vi "Stop Acquisition.vi"(8 "error in (no error)":errorcluster, 11 "Hardware Resources in":T1={"VISA Refnum in"="", "Serial Configuration"={"Baud Rate"=460800, "Flow Control"=0}, "Voltage Level (0V)"=0.0, "Output Phase(s) (1-Phase)"=0, "Active Phase (1:Phase 1)"=1} {"Output Phase(s) (1-Phase)" items=["3 phase", "1 phase"]; "Active Phase (1:Phase 1)" items=["Phase 1"=1, "Phase 2"=2, "Phase 3"=3]; "Serial Configuration"."Flow Control" items=["None", "XON/XOFF", "RTS/CTS", "XON/XOFF & RTS/CTS", "DTR/DSR", "XON/XOFF & DTR/DSR"]; "Serial Configuration"."Baud Rate" items=["9600"=9600, "19200"=19200, "38400"=38400, "57600"=57600, "115200"=115200, "230400"=230400, "460800"=460800]}) -> (0 "error out":errorcluster)   [LabVIEW 2013, in "Cal Inst Acquisition.lvlib"]
doc: "Stops the acquisition."
uses:
  Cal Inst Acquisition.lvlib
  Hardware Configuration.ctl
  Libraries/California Instruments iX Series/California Instruments iX Series.lvlib
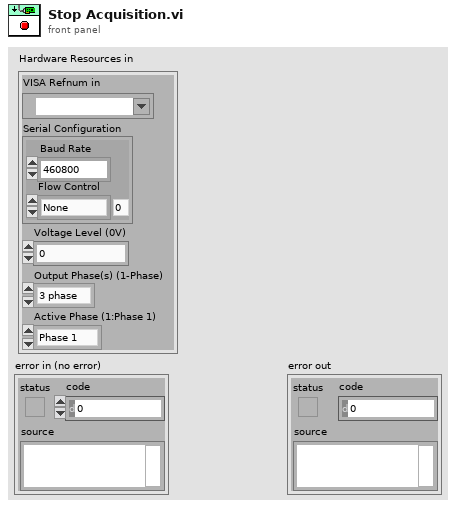
[diagram p1: front panel]
types:
  T1 = typedef "Cal Inst Acquisition.lvlib/Hardware Configuration.ctl" = cluster{"VISA Refnum in":refnum<visa-resource-name>, "Serial Configuration":cluster{"Baud Rate":u32, "Flow Control":u16}, "Voltage Level (0V)":dbl, "Output Phase(s) (1-Phase)":u16, "Active Phase (1:Phase 1)":i32}
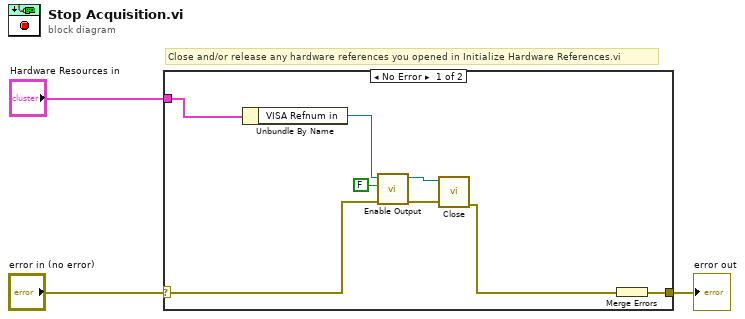
[diagram p0: block diagram]
diagram:
  # "Close and/or release any hardware references you opened in Initialize Hardware References.vi"
  n1 = case shown="No Error" "error in (no error)" {
    selector: "error in (no error)" -> [w5 w12]
    tunnel: [w11 w12] -> w2
    tunnel: "Hardware Resources in" -> [w10 _]
    frame No Error {
      n2 = Unbundle By Name(w10) -> ("VISA Refnum in"=w6:refnum<visa-resource-name>)
      n3 = call "Enable Output.vi"("error in (no error)"=w5, "Enable Output (T: Enable)"=FALSE, "VISA resource name"=w6) -> ("error out"=w8:errorcluster, "VISA resource name out"=w7:refnum<visa-resource-name>)  [unwired: 7 in]
      n4 = call "Close.vi"("error in (no error)"=w8, "VISA resource name"=w7) -> ("error out"=w4:errorcluster)  [unwired: 9 in]
      n5 = Merge Errors(w4) -> (w11:errorcluster)
    }
    frame Error {
    }
  }
  "error out" <- w2
